vi "Pawn_Init.vi"(8 "error in (no error)":errorcluster, 11 "Object in":refnum<class "Pawn.lvclass">) -> (0 "error out":errorcluster, 3 "object out":refnum<class "Pawn.lvclass">)   [LabVIEW 2020]
uses:
  Pawn.lvclass
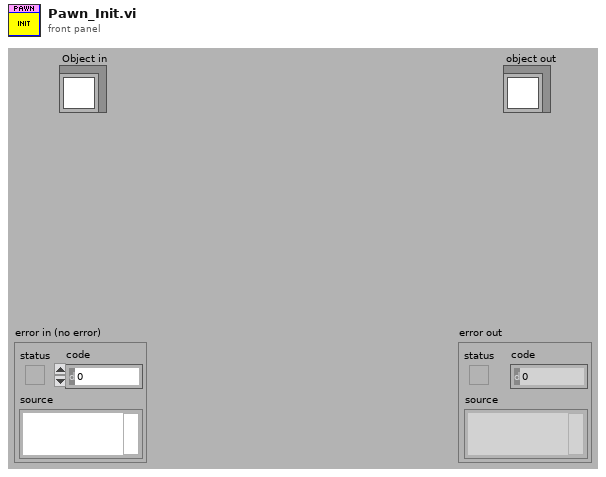
[diagram p1: front panel]
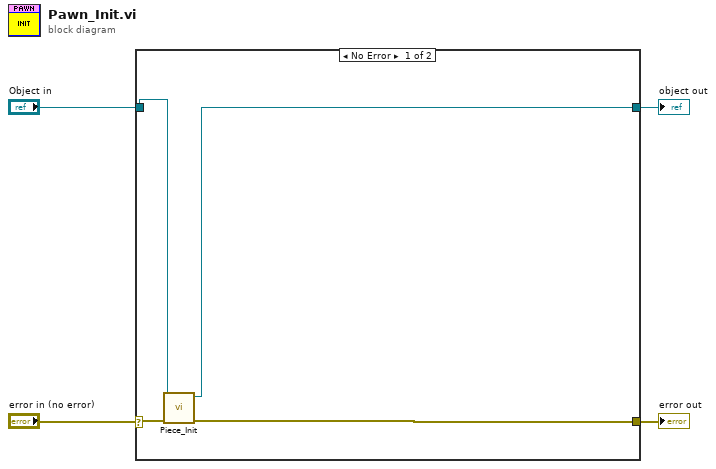
[diagram p0: block diagram]
diagram:
  n1 = case shown="No Error" "error in (no error)" {
    selector: "error in (no error)" -> [w8 w9]
    tunnel: [w5 w10] -> w4
    tunnel: "Object in" -> [w6 w10]
    tunnel: [w7 w9] -> w1
    frame No Error {
      n2 = call-dynamic "Piece_Init.vi"("error in (no error)"=w8, "object in"=w6) -> ("error out"=w7:errorcluster, "object out"=w5:refnum<class "Pawn.lvclass">)  [unwired: 8 in]
    }
    frame Error {
    }
  }
  "object out" <- w4
  "error out" <- w1
